vi "Check Static Pressure.vi"(8 "error in (no error)":errorcluster, 10 "Set P ATM? (F)":bool, 11 "BaseProducer in":refnum<class "BaseProducer.lvclass">) -> (0 "error out":errorcluster, 2 "Pressure (psi atm)":dbl, 3 "BaseProducer out":refnum<class "BaseProducer.lvclass">)   [LabVIEW 2013, in "BaseProducer.lvclass"]
doc: "This method reads the static pressure sensor value, converts it to psi abs, and sets this object's atmospheric pressure value accordingly."
uses:
  BaseProducer.lvclass
  BaseProducer.lvclass/BaseProducer.ctl
  <vilib>/DAQmx/read.llb/DAQmx Read (Analog 1D DBL NChan 1Samp).vi
  <vilib>/DAQmx/miscellaneous.llb/DAQmx Fill In Error Info.vi
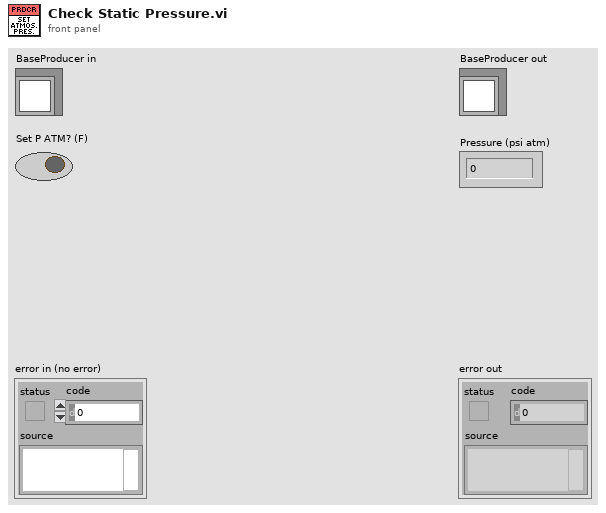
[diagram p1: front panel]
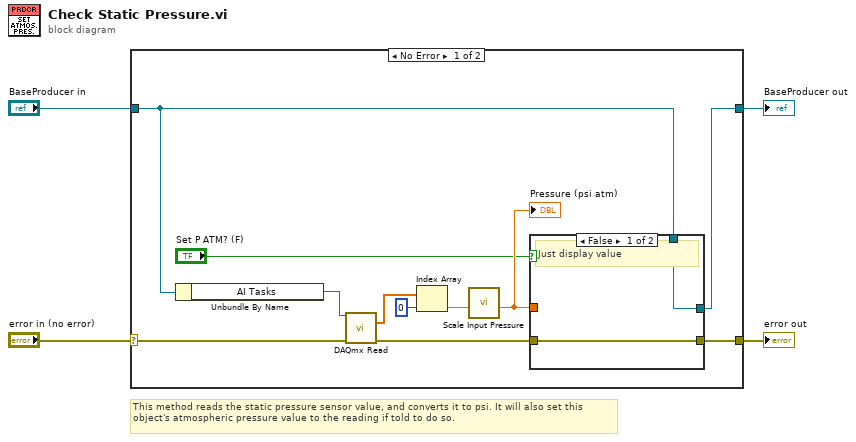
[diagram p0: block diagram]
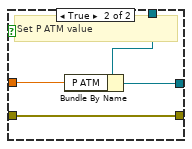
[diagram p2: hidden frame]
diagram:
  # "This method reads the static pressure sensor value, and converts it to psi. It will also set this object's atmospheric pressure value to the reading if told to do so."
  n1 = case shown="No Error" "error in (no error)" {
    selector: "error in (no error)" -> [w15 w23]
    tunnel: [w5 w23] -> w3
    tunnel: [w7 w22] -> w1
    tunnel: "BaseProducer in" -> [w10 w22]
    frame No Error {
      n2 = Unbundle By Name(w10) -> ("AI Tasks"=w14:refnum<k21>)
      n3 = call-poly <vilib>:"DAQmx Read.vi"("task/channels in"=w14, "error in"=w15) -> ("data"=w13:dbl[], "error out"=w9:errorcluster)  [unwired: 11 in, 1 out]
      n4 = Index Array(array=w13, index=0) -> (element=w11:dbl)
      n5 = call "Scale Input Pressure.vi"("Pressure (V)"=w11) -> ("Pressure (psi atm)"=w8:dbl)  [unwired: 10 in]
      "Pressure (psi atm)" <- w8
      n6 = case shown="False" "Set P ATM? (F)" {
        tunnel: w10 -> [w17 w21]
        tunnel: w9 -> [w16 w18]
        tunnel: w8 -> [_ w20]
        tunnel: [w17 w19] -> w7
        tunnel: [w16 w18] -> w5
        frame False {
          # "Just display value"
        }
        frame True {
          # "Set P ATM value"
          n7 = Bundle By Name(cluster=w21, "P ATM"=w20) -> (w19:refnum<class "BaseProducer.lvclass">)
        }
      }
    }
    frame Error {
    }
  }
  "error out" <- w3
  "BaseProducer out" <- w1
